vi "Actor Core.vi"(8 "Error in":errorcluster, 11 "UI in":refnum<class "UI.lvclass">) -> (0 "Error out":errorcluster, 3 "Actor out":refnum<class "Actor.lvclass">)   [LabVIEW 2016, in "UI.lvlib" / "UI.lvclass"]
doc: "This VI will help in understanding the basic image processing techniques"
uses:
  UI.lvclass
  <vilib>/userdefined/High Color/IMAQdx.ctl
  C:/Program Files (x86)/National Instruments/LabVIEW 2016/vi.lib/ActorFramework/Actor/Actor.lvclass
  <vilib>/ActorFramework/Actor/Actor.lvclass
  Controls/UI States.ctl
  Controls/Data.ctl
  <vilib>/ActorFramework/Message Enqueuer/Message Enqueuer.lvclass
  UI.lvclass/UI.ctl
  <vilib>/vision/Image Controls.llb/IMAQ Image.ctl
  <vilib>/ActorFramework/Actor/Actor.lvclass/Actor.ctl
  <vilib>/ActorFramework/Message Enqueuer/Message Enqueuer.lvclass/Message Enqueuer.ctl
  Controls/Start Acquisition.ctl
  Controller/Controller Messages/Acquistion Request Msg/Acquistion Request Msg.lvclass/Acquistion Request Msg.ctl
  <vilib>/ActorFramework/Report Error Msg/Report Error Msg.lvclass/Report Error Msg.ctl
  <vilib>/ActorFramework/Message Enqueuer/Init from Existing Queue.vi
  <vilib>/ActorFramework/Message Enqueuer/Enqueue.vi
  Controller/Controller Messages/Stop Controller Msg/Stop Controller Msg.lvclass
  C:/Program Files (x86)/National Instruments/LabVIEW 2016/vi.lib/ActorFramework/Message/Message.lvclass
  Controller/Controller Messages/Acquistion Request Msg/Acquistion Request Msg.lvclass
  Controller/Controller Messages/Stop Acquistion Msg/Stop Acquistion Msg.lvclass
  Controller/Controller Messages/Launch Grayscale Msg/Launch Grayscale Msg.lvclass
  Controller/Controller Messages/Launch Histogram Msg/Launch Histogram Msg.lvclass
  Controller/Controller Messages/Launch Threshold Msg/Launch Threshold Msg.lvclass
  <vilib>/ActorFramework/Report Error Msg/Report Error Msg.lvclass
  <vilib>/ActorFramework/Stop Msg/Stop Msg.lvclass
  <vilib>/ActorFramework/Message Priority Queue/Priority Enqueue.vi
panel:
  in  "Help Button":bool
  in  "Launch Threshold":bool
  in  "Launch Histogram":bool
  in  "Launch Grayscale":bool
  in  "Stop Acquisition":bool
  in  "Start Acquisition":bool
  in  "Choose Camera":T1
  out "Live Feed":T2(plugin-control)
  # "Image Analyzer"
  # "Operations Available"
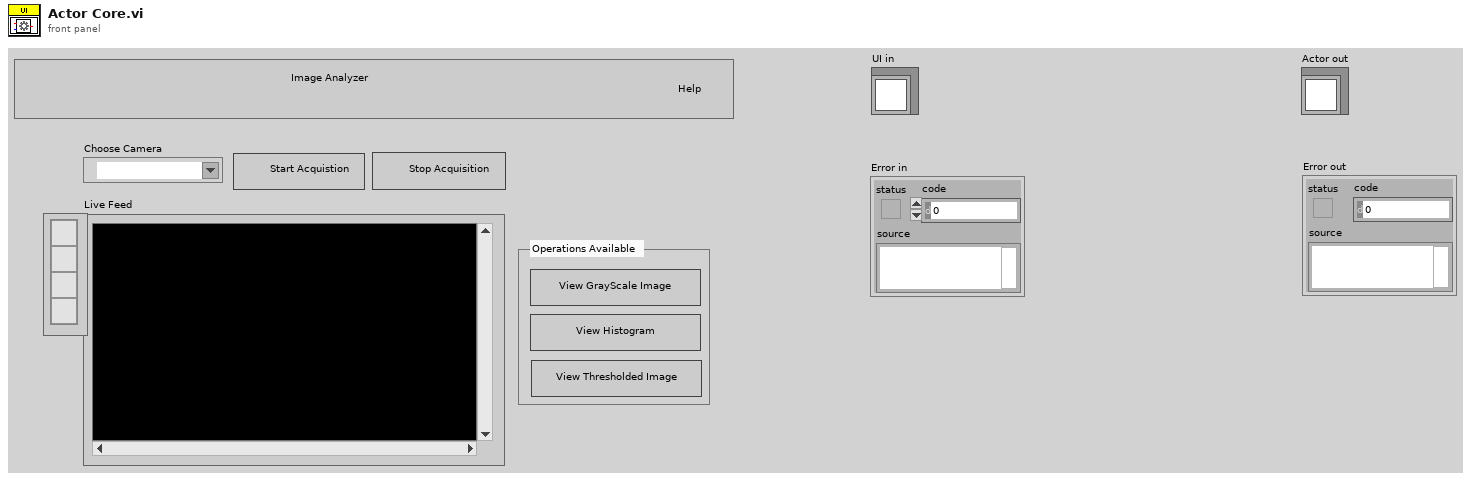
[diagram p1: front panel]
types:
  T1 = typedef "IMAQdx.ctl" = refnum<k21>
  T2 = typedef "IMAQ Image.ctl" = refnum<image>
  T3 = typedef "Data.ctl" = cluster{"UI in":refnum<class "UI.lvclass">, "Self Enqueuer":refnum<class "Message Enqueuer.lvclass">, "AcquistionActorEnqueuer":refnum<class "Message Enqueuer.lvclass">, "Caller Enqueuer":refnum<class "Message Enqueuer.lvclass">, "Event Reg Refnum":refnum<event-registration>}
  T4 = typedef "UI States.ctl" = enum16{"Poll UI", "Initialize", "Start Acquisition", "Stop Acquisition", "Launch Grayscale", "LaunchHistogram", "LaunchThreshold", "Error", "Exit"}
  T5 = enum8{"Enabled", "Disabled", "Disabled and Grayed Out"}
  T6 = typedef "Start Acquisition.ctl" = cluster{"Image Indicator Reference":refnum<vi>, "Start":bool, "Camera":T1}
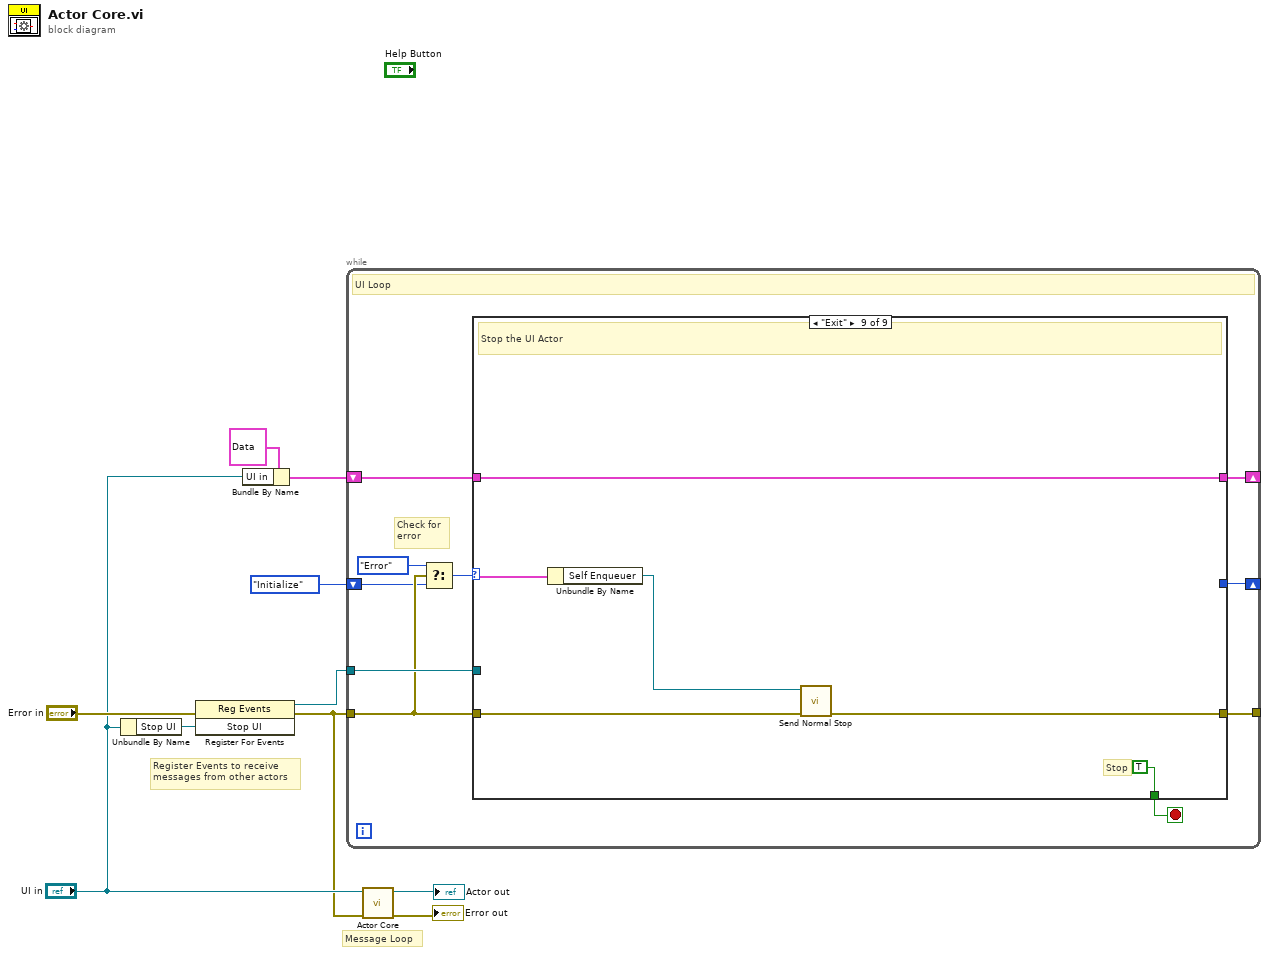
[diagram p0: block diagram]
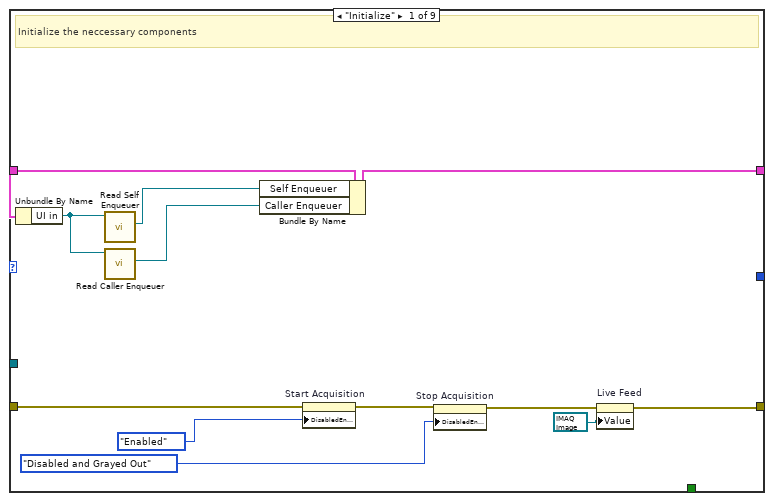
[diagram p2: hidden frame]
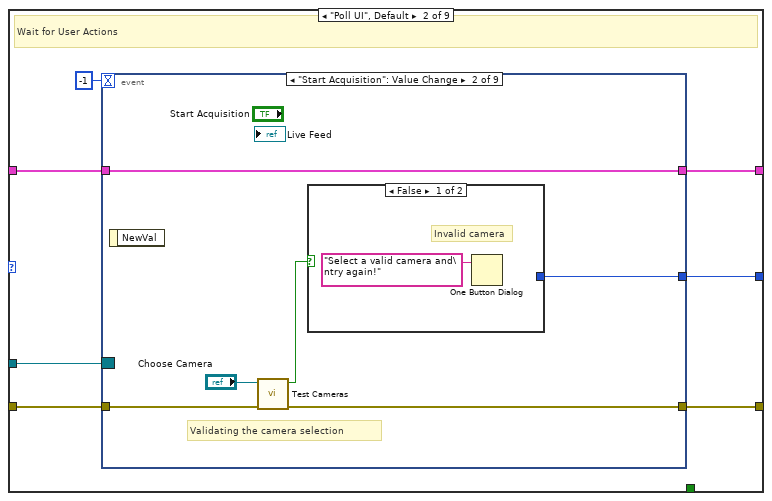
[diagram p3: hidden frame]
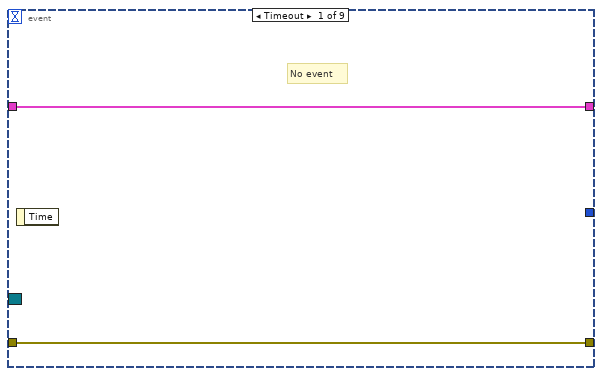
[diagram p4: hidden frame]
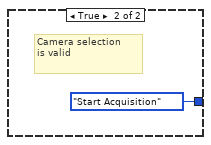
[diagram p5: hidden frame]
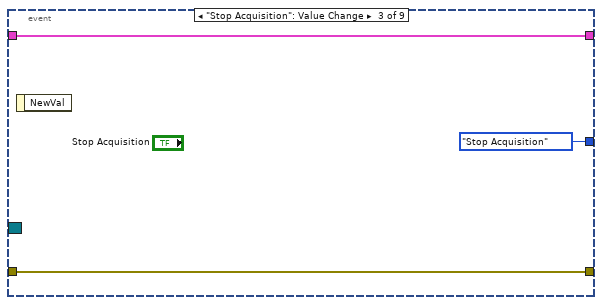
[diagram p6: hidden frame]
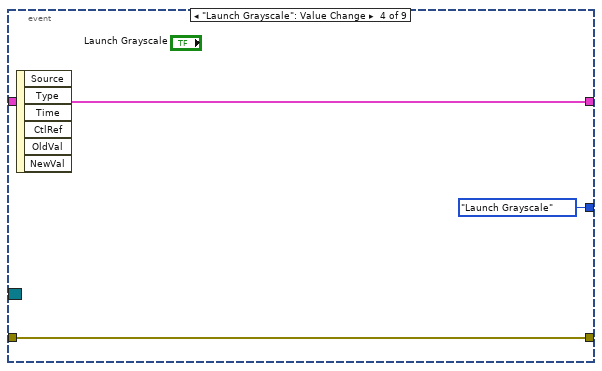
[diagram p7: hidden frame]
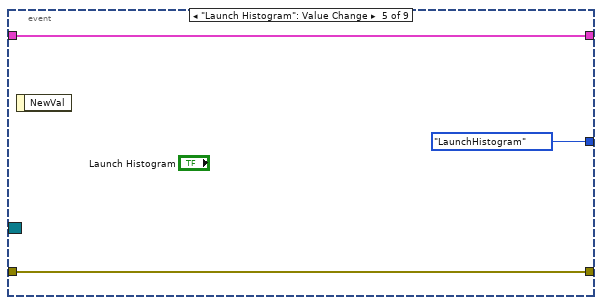
[diagram p8: hidden frame]
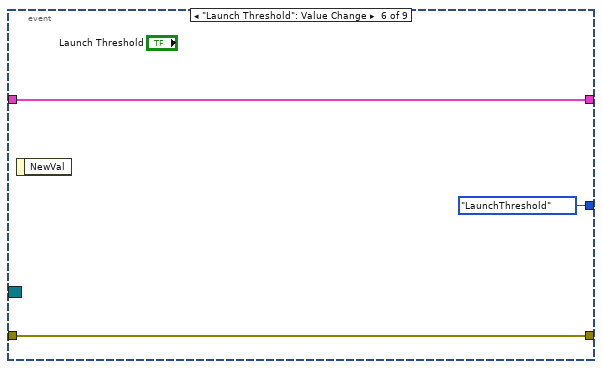
[diagram p9: hidden frame]
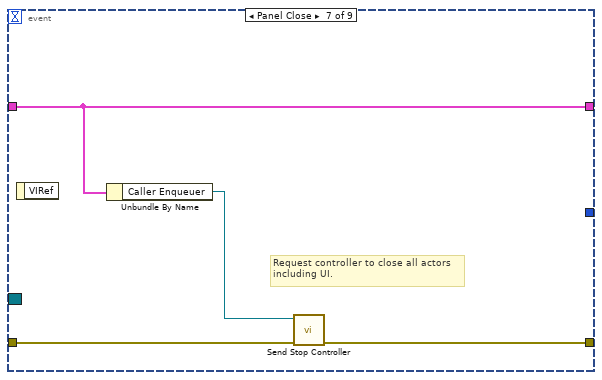
[diagram p10: hidden frame]
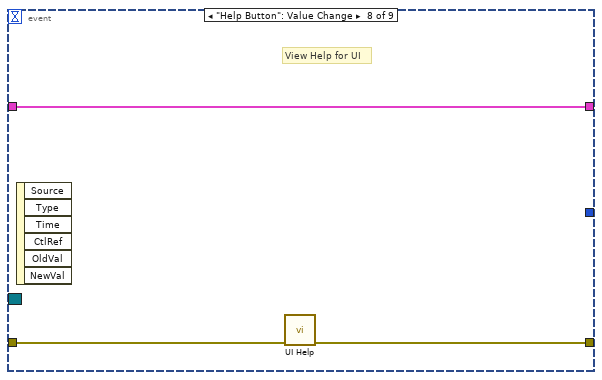
[diagram p11: hidden frame]
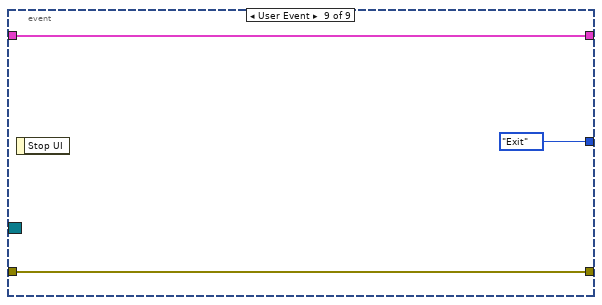
[diagram p12: hidden frame]
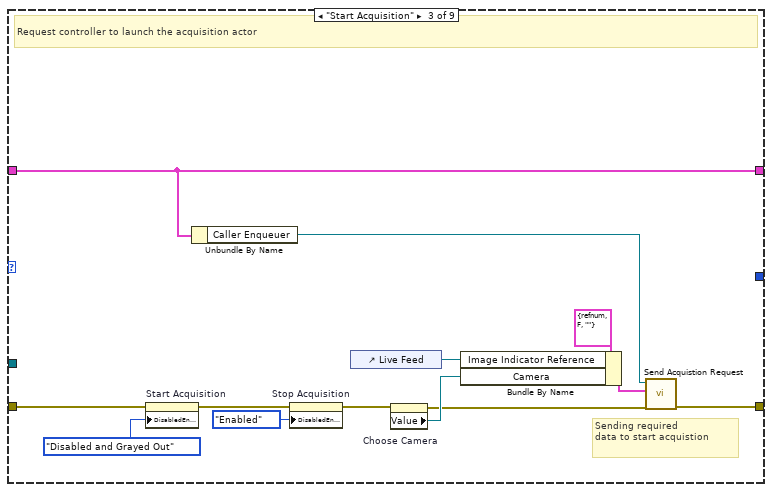
[diagram p13: hidden frame]
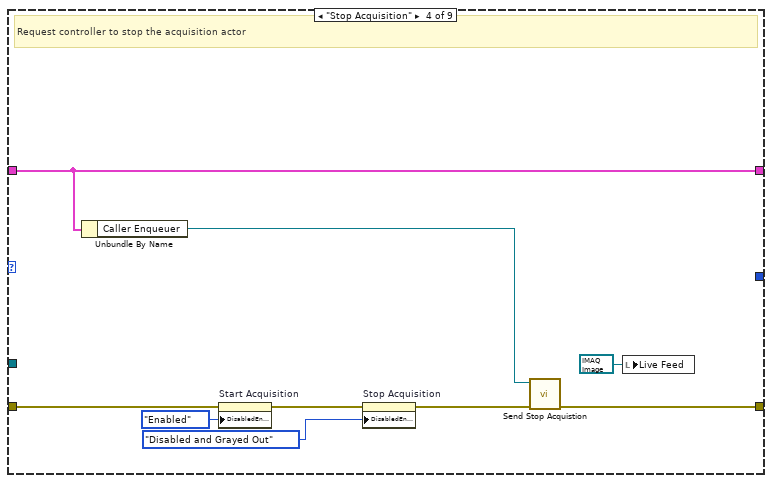
[diagram p14: hidden frame]
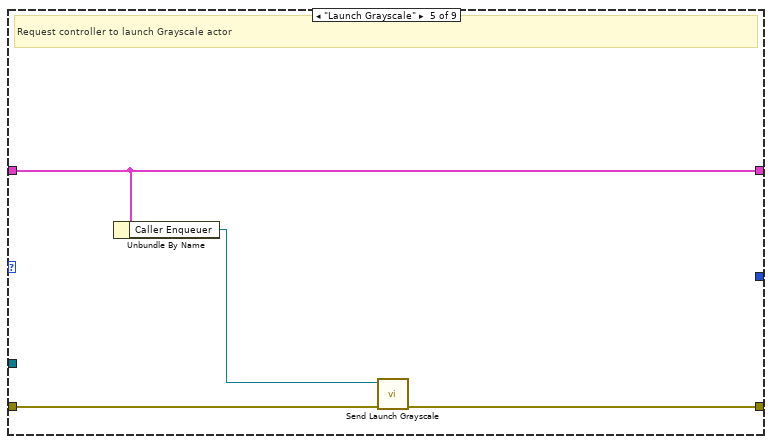
[diagram p15: hidden frame]
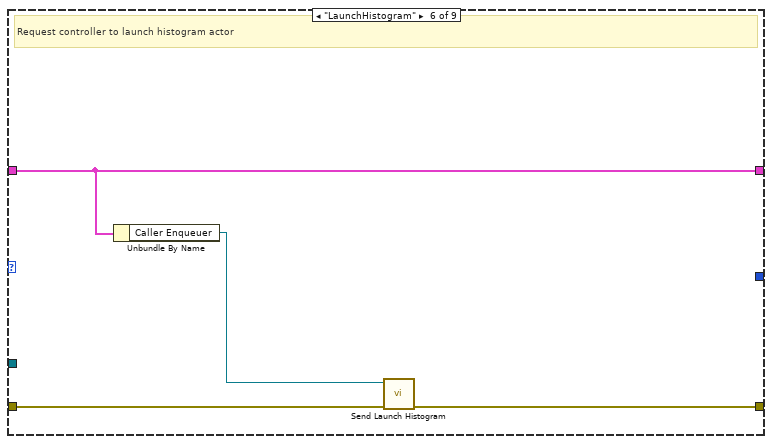
[diagram p16: hidden frame]
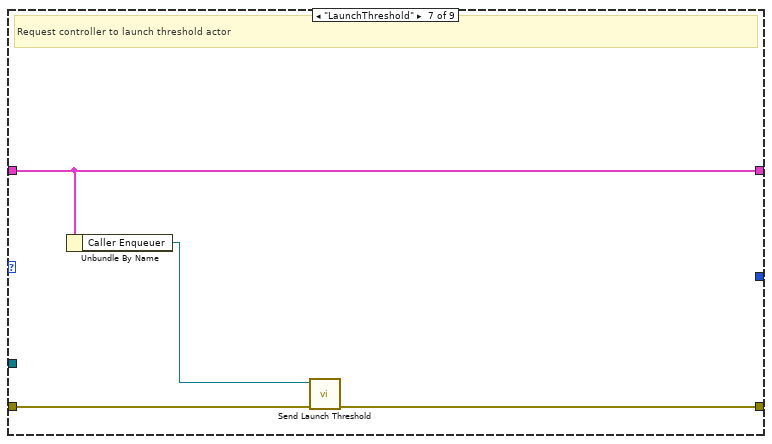
[diagram p17: hidden frame]
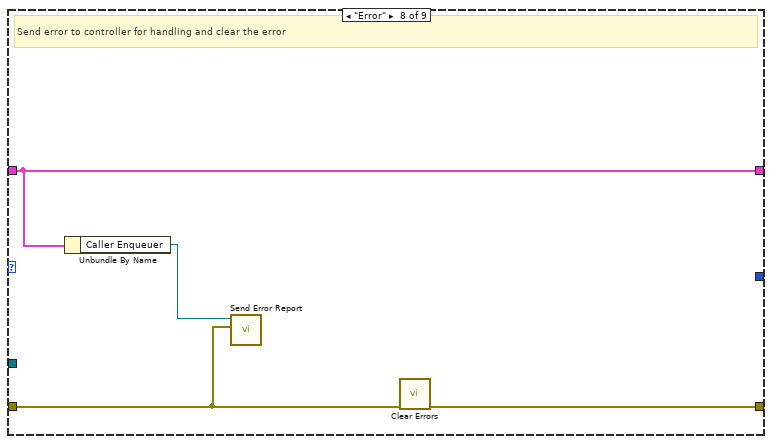
[diagram p18: hidden frame]
diagram:
  # "Message Loop"
  # "Register Events to receive\nmessages from other actors"
  n1 = Unbundle By Name("UI in") -> ("Stop UI"=w5:refnum<user-event>)
  n2 = register-events(error in="Error in", w5) -> (reference out=w2:refnum<event-registration>, error out=w1:errorcluster)  [unwired: 1 in]
  n3 = Bundle By Name(cluster=T3 {"UI in"=refnum, "Self Enqueuer"=refnum, "AcquistionActorEnqueuer"=refnum, "Caller Enqueuer"=refnum, "Event Reg Refnum"=refnum}, "UI in"="UI in") -> (w6:T3)
  n4 = while {
    shift-right: [w18] -> _
    shift-left: UI_States."Initialize" -> [w12]
    tunnel: w1 -> [w14]
    shift-right: [w16] -> _
    shift-left: w6 -> [w20]
    tunnel: [w19] -> _
    tunnel: w2 -> [w15]
    stop <- w17 stop-if-true
    # "Check for\nerror"
    # "UI Loop"
    n5 = Select(t=UI_States."Error", s=w14, f=w12) -> (s? t:f=w11:T4)
    n6 = case shown="\"Exit\"" w11 {
      tunnel: w20 -> [w31 w39 w79 w92 w95 w99 w103 w109 w113]
      tunnel: w14 -> [w24 w38 w77 w88 w97 w101 w105 w107 w112]
      tunnel: [w21 w37 w81 w93 w96 w100 w104 w106 w111] -> w19
      tunnel: [_ w36 _ _ _ _ _ _ _] -> w18
      tunnel: [_ _ _ _ _ _ _ _ TRUE] -> w17
      tunnel: [w32 w35 w79 w92 w95 w99 w103 w109 w113] -> w16
      tunnel: w15 -> [_ w34 _ _ _ _ _ _ _]
      frame "Initialize" {
        # "Initialize the neccessary components"
        n7 = Unbundle By Name(w31) -> ("UI in"=w30:refnum<class "UI.lvclass">)
        n8 = call <vilib>:"Read Self Enqueuer.vi"("Actor"=w30) -> ("Self Enqueuer"=w29:refnum<class "Message Enqueuer.lvclass">)  [unwired: 10 in]
        n9 = call <vilib>:"Read Caller Enqueuer.vi"("Actor"=w30) -> ("Caller Enqueuer"=w28:refnum<class "Message Enqueuer.lvclass">)  [unwired: 10 in]
        n10 = Bundle By Name(cluster=w31, "Self Enqueuer"=w29, "Caller Enqueuer"=w28) -> (w32:T3)
        n11 = property on="Start Acquisition" class="Bool"(error in=w24, "DisabledEnum"=T5."Enabled" ("Disabled")) -> (error out=w25:errorcluster)  [unwired: 1 in, 1 out]
        n12 = property on="Stop Acquisition" class="Bool"(error in=w25, "DisabledEnum"=T5."Disabled and Grayed Out" ("Disabled")) -> (error out=w22:errorcluster)  [unwired: 1 in, 1 out]
        n13 = property on="Live Feed" class="ImageControl"(error in=w22, "Value"=T2 refnum ("Live Feed")) -> (error out=w21:errorcluster)  [unwired: 1 in, 1 out]
      }
      frame "Poll UI", Default {
        # "Wait for User Actions"
        n14 = event shown="[1] \"Start Acquisition\": Value Change" {
          selector: w34 -> [_ _ _ _ _ _ _ _ _]
          dyn-events: _ -> [_ _ _ _ _ _ _ _ _]
          timeout: -1 -> [_ _ _ _ _ _ _ _ _]
          tunnel: w39 -> [w40 w47 w51 w54 w57 w60 w65 w68 w70]
          tunnel: w38 -> [w41 w46 w52 w55 w58 w61 w63 w67 w71]
          tunnel: [w41 w45 w52 w55 w58 w61 w62 w66 w71] -> w37
          tunnel: [_ w43 UI_States."Stop Acquisition" UI_States."Launch Grayscale" UI_States."LaunchHistogram" UI_States."LaunchThreshold" _ _ UI_States."Exit"] -> w36
          tunnel: [w40 w47 w51 w54 w57 w60 w65 w68 w70] -> w35
          event Timeout {
            # "No event"
            n15 = event-data() -> ()  [unwired: 1 in, 1 out]
          }
          event "Start Acquisition": Value Change {
            # "Validating the camera selection"
            n16 = event-data() -> ()  [unwired: 1 in, 1 out]
            n17 = call "Test Cameras.vi"("error in"=w46, "Session In"="Choose Camera") -> ("error out"=w45:errorcluster, "Valid Camera"=w44:bool)  [unwired: 8 in]
            n18 = case shown="False" w44 {
              tunnel: [_ UI_States."Start Acquisition"] -> w43
              frame False {
                # "Invalid camera"
                n19 = One Button Dialog(message="Select a valid camera and\ntry again!") -> ()  [unwired: 1 in, 1 out]
              }
              frame True {
                # "Camera selection\nis valid"
              }
            }
          }
          event "Stop Acquisition": Value Change {
            n20 = event-data() -> ()  [unwired: 1 in, 1 out]
          }
          event "Launch Grayscale": Value Change {
            n21 = event-data() -> ()  [unwired: 1 in, 6 out]
          }
          event "Launch Histogram": Value Change {
            n22 = event-data() -> ()  [unwired: 1 in, 1 out]
          }
          event "Launch Threshold": Value Change {
            n23 = event-data() -> ()  [unwired: 1 in, 1 out]
          }
          event Panel Close {
            # "Request controller to close all actors\nincluding UI."
            n24 = event-data() -> ()  [unwired: 1 in, 1 out]
            n25 = Unbundle By Name(w65) -> ("Caller Enqueuer"=w64:refnum<class "Message Enqueuer.lvclass">)
            n26 = call "Send Stop Controller.vi"("error in (no error)"=w63, "Message Enqueuer"=w64) -> ("error out"=w62:errorcluster)  [unwired: 8 in, 1 out]
          }
          event "Help Button": Value Change {
            # "View Help for UI"
            n27 = event-data() -> ()  [unwired: 1 in, 6 out]
            n28 = call "UI Help.vi"("error in (no error)"=w67) -> ("error out"=w66:errorcluster)  [unwired: 10 in]
          }
          event User Event {
            n29 = event-data() -> ()  [unwired: 1 in, 1 out]
          }
        }
      }
      frame "Start Acquisition" {
        # "Sending required\ndata to start acquistion"
        # "Request controller to launch the acquisition actor"
        n30 = property on="Start Acquisition" class="Bool"(error in=w77, "DisabledEnum"=T5."Disabled and Grayed Out" ("Disabled")) -> (error out=w75:errorcluster)  [unwired: 1 in, 1 out]
        n31 = Unbundle By Name(w79) -> ("Caller Enqueuer"=w80:refnum<class "Message Enqueuer.lvclass">)
        n32 = property on="Stop Acquisition" class="Bool"(error in=w75, "DisabledEnum"=T5."Enabled" ("Disabled")) -> (error out=w73:errorcluster)  [unwired: 1 in, 1 out]
        n33 = control-ref of="Live Feed"() -> (w82:refnum<vi>)
        n34 = property on="Choose Camera" class="IMAQdx (strict)"(error in=w73) -> (error out=w72:errorcluster, "Value"=w78:T1)  [unwired: 1 in, 1 out]
        n35 = Bundle By Name(cluster=T6 {"Image Indicator Reference"=refnum, "Start"=FALSE, "Camera"=""} ("Start Acquisition"), "Image Indicator Reference"=w82, "Camera"=w78) -> (w83:T6)
        n36 = call "Send Acquistion Request.vi"("error in (no error)"=w72, "Start Acquisition"=w83, "Message Enqueuer"=w80) -> ("error out"=w81:errorcluster)  [unwired: 7 in, 1 out]
      }
      frame "Stop Acquisition" {
        # "Request controller to stop the acquisition actor"
        n37 = Unbundle By Name(w92) -> ("Caller Enqueuer"=w91:refnum<class "Message Enqueuer.lvclass">)
        n38 = property on="Start Acquisition" class="Bool"(error in=w88, "DisabledEnum"=T5."Enabled" ("Disabled")) -> (error out=w87:errorcluster)  [unwired: 1 in, 1 out]
        n39 = property on="Stop Acquisition" class="Bool"(error in=w87, "DisabledEnum"=T5."Disabled and Grayed Out" ("Disabled")) -> (error out=w86:errorcluster)  [unwired: 1 in, 1 out]
        n40 = call "Send Stop Acquistion.vi"("error in (no error)"=w86, "Message Enqueuer"=w91) -> ("error out"=w93:errorcluster)  [unwired: 8 in, 1 out]
        n41 = local write "Live Feed"(T2 refnum ("Live Feed")) -> ()
      }
      frame "Launch Grayscale" {
        # "Request controller to launch Grayscale actor"
        n42 = Unbundle By Name(w95) -> ("Caller Enqueuer"=w94:refnum<class "Message Enqueuer.lvclass">)
        n43 = call "Send Launch Grayscale.vi"("error in (no error)"=w97, "Message Enqueuer"=w94) -> ("error out"=w96:errorcluster)  [unwired: 8 in, 1 out]
      }
      frame "LaunchHistogram" {
        # "Request controller to launch histogram actor"
        n44 = Unbundle By Name(w99) -> ("Caller Enqueuer"=w98:refnum<class "Message Enqueuer.lvclass">)
        n45 = call "Send Launch Histogram.vi"("error in (no error)"=w101, "Message Enqueuer"=w98) -> ("error out"=w100:errorcluster)  [unwired: 8 in, 1 out]
      }
      frame "LaunchThreshold" {
        # "Request controller to launch threshold actor"
        n46 = Unbundle By Name(w103) -> ("Caller Enqueuer"=w102:refnum<class "Message Enqueuer.lvclass">)
        n47 = call "Send Launch Threshold.vi"("error in (no error)"=w105, "Message Enqueuer"=w102) -> ("error out"=w104:errorcluster)  [unwired: 8 in, 1 out]
      }
      frame "Error" {
        # "Send error to controller for handling and clear the error"
        n48 = Unbundle By Name(w109) -> ("Caller Enqueuer"=w108:refnum<class "Message Enqueuer.lvclass">)
        n49 = call <vilib>:"Send Error Report.vi"("Error From Sender"=w107, "Message Enqueuer"=w108) -> ()  [unwired: 9 in, 1 out]
        n50 = call <vilib>:"Clear Errors.vi"("error in (no error)"=w107) -> ("error out"=w106:errorcluster)  [unwired: 5 in, 1 out]
      }
      frame "Exit" {
        # "Stop"
        # "Stop the UI Actor"
        n51 = Unbundle By Name(w113) -> ("Self Enqueuer"=w110:refnum<class "Message Enqueuer.lvclass">)
        n52 = call <vilib>:"Send Normal Stop.vi"("error in (no error)"=w112, "Message Enqueuer"=w110) -> ("error out"=w111:errorcluster)  [unwired: 9 in]
      }
    }
  }
  n53 = call-parent "Actor Core.vi"("error in"=w1, "Actor in"="UI in") -> ("error out"=→"Error out":errorcluster, "Actor out"=→"Actor out":refnum<class "Actor.lvclass">)  [unwired: 8 in]
